vi "Write On End Message.vi"(8 "error in (no error)":errorcluster, 10 "Actor Framework:Message":refnum<class "Message.lvclass">, 11 "Replay Msg in":refnum<class "Replay Msg.lvclass">) -> (0 "error out":errorcluster, 3 "Replay Msg out":refnum<class "Replay Msg.lvclass">)   [LabVIEW 2014, in "Replay Msg.lvclass"]
uses:
  ExperimentService/Replay Msg.lvclass
  <vilib>/ActorFramework/Message/Message.lvclass
  ExperimentService/Replay Msg.lvclass/Replay Msg.ctl
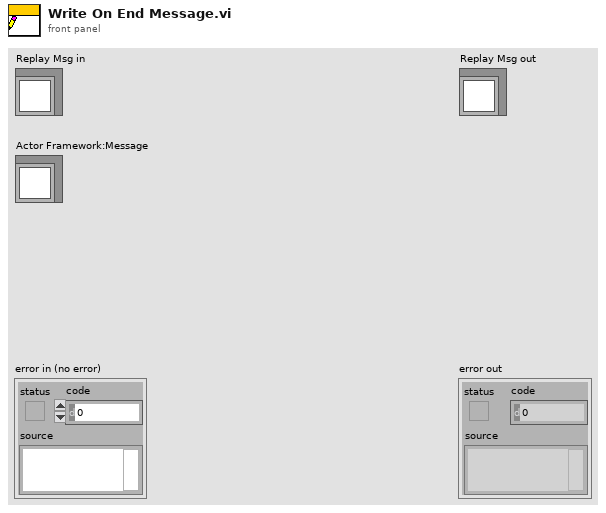
[diagram p1: front panel]
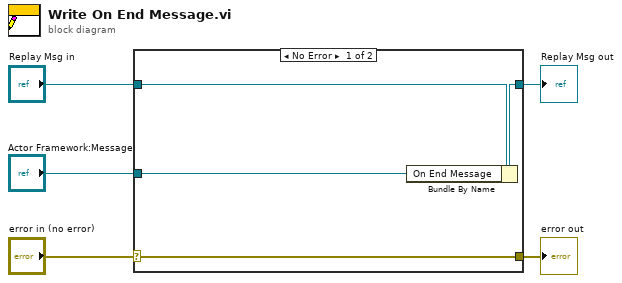
[diagram p0: block diagram]
diagram:
  n1 = case shown="No Error" "error in (no error)" {
    selector: "error in (no error)" -> [w9 w10]
    tunnel: [w9 w10] -> w4
    tunnel: [w7 w11] -> w2
    tunnel: "Replay Msg in" -> [w8 w11]
    tunnel: "Actor Framework:Message" -> [w6 _]
    frame No Error {
      n2 = Bundle By Name(cluster=w8, "On End Message"=w6) -> (w7:refnum<class "Replay Msg.lvclass">)
    }
    frame Error {
    }
  }
  "error out" <- w4
  "Replay Msg out" <- w2
